vi "BEO Winkelgeschwindigkeit.vi"(8 "Kraft (N)":dbl, 9 "Ist-Zustand Position (m, m/s)":cluster{"Position":dbl, "Geschwindigkeit":dbl}, 10 "Winkel (rad)":T2) -> (3 "Winkelgeschwindigkeit (1/s)":T1)   [LabVIEW 2014]
uses:
  <vilib>/Simulation/Scripting/Companion Diagram/SimConfigNode/SimParams.ctl
  <vilib>/Simulation/Scripting/Companion Diagram/SimConfigNode/_simSolvers.ctl
  <vilib>/Simulation/Implementation/Shared/SIMSCR Execution Mode.ctl
  <vilib>/Simulation/Param Hierarchy/Typedefs/SIMPH Param Control Actions.ctl
  <vilib>/Simulation/Implementation/Shared/NILVSim_ParamChanged.vi
  <vilib>/Simulation/Implementation/Shared/NILVSIM_BeginStep.vi
  <vilib>/Simulation/Implementation/Shared/NILVSim_Manager.vi
  <vilib>/Utility/error.llb/Clear Errors.vi
  <vilib>/Simulation/Implementation/Shared/NILVSim_FinalizeModel.vi
  <vilib>/Simulation/Implementation/Shared/SIM Unbundle Sim Info.vi
  <vilib>/Simulation/Implementation/Shared/NILVSim_Initialize.vi
  <vilib>/Simulation/Utility/Implementation/NILVSim Get Time and IsAcceptedStep.vi
  <vilib>/Simulation/Implementation/Shared/SIMSH Read Queue.vi
  <vilib>/Simulation/Implementation/Shared/NILVSim_GetModelError.vi
  <vilib>/Simulation/Implementation/Shared/SIM Bundle Sim Info.vi
  <vilib>/Simulation/Implementation/XNodeFramework/SimXNode/SimX.xnode
  Beobachter/Nichtlinearer Beobachter.vi
  <vilib>/Simulation/Scripting/Companion Diagram/SimConfigNode/SimDog.xnode
  <vilib>/Simulation/Implementation/Shared/NI_SIM_Implementation.lvlib
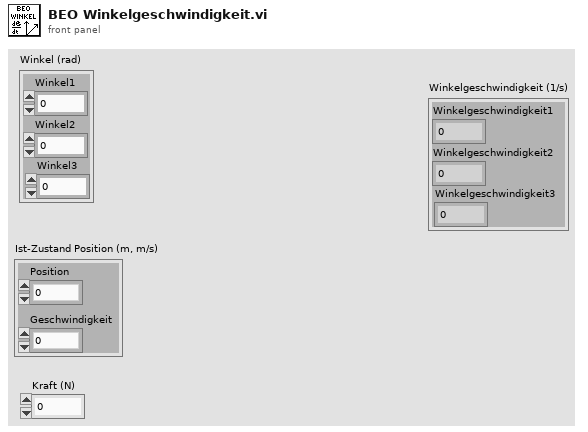
[diagram p1: front panel]
types:
  T1 = cluster{"Winkelgeschwindigkeit1":dbl, "Winkelgeschwindigkeit2":dbl, "Winkelgeschwindigkeit3":dbl}
  T2 = cluster{"Winkel1":dbl, "Winkel2":dbl, "Winkel3":dbl}
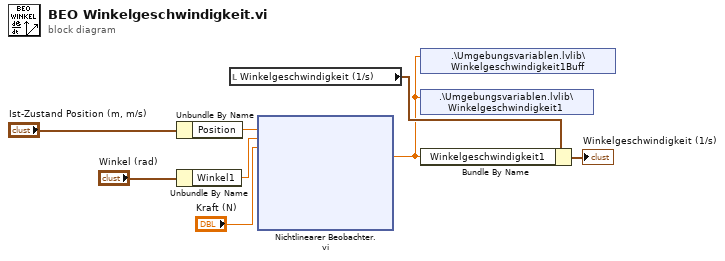
[diagram p0: block diagram]
diagram:
  n1 = Unbundle By Name("Ist-Zustand Position (m, m/s)") -> ("Position"=w4:dbl)
  n2 = Unbundle By Name("Winkel (rad)") -> ("Winkel1"=w3:dbl)
  n3 = local read "Winkelgeschwindigkeit (1/s)"() -> (w7:T1)
  n4 = xnode "Nichtlinearer Beobachter.vi"("x1"=w4, "x3"=w3, "u"="Kraft (N)") -> ("x4_"=w1:dbl)  [unwired: 2 in, 25 out]
  n5 = shared-variable ".\\Umgebungsvariablen.lvlib\\Winkelgeschwindigkeit1Buff"(w1) -> ()  [unwired: 1 in, 1 out]
  n6 = shared-variable ".\\Umgebungsvariablen.lvlib\\Winkelgeschwindigkeit1"(w1) -> ()  [unwired: 1 in, 1 out]
  n7 = Bundle By Name(cluster=w7, "Winkelgeschwindigkeit1"=w1) -> (→"Winkelgeschwindigkeit (1/s)":T1)
